vi "Datalog Evaluator.vi"(5 "LuaVIEW reference":T1) -> (15 "error out":errorcluster)   [LabVIEW 2012]
doc: "This plug-in is required by the \"datalogging\" runlevel. It performs tag expression evaluation updates."
uses:
  luaview/typedefs/t_LuaVIEW Reference.ctl
  typedefs/t_Datalog Periodic Evaluator States.ctl
  typedefs/t_DataLog Expression Update Timing Methods.ctl
  typedefs/t_DataLog Tag Info List Methods.ctl
  typedefs/t_DataLog Tag Expression Evaluator Methods.ctl
  luaview/typedefs/t_LuaVIEW Task State Methods.ctl
  luaview/subvis/private/LuaVIEW Pull (flat data).vi
  subvis/private/glb_DataLog Runtime Parameterisation.vi
panel:
  in  "default config":cluster{"tag expression definitions":string}
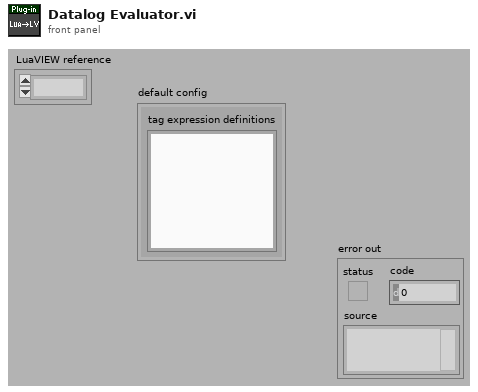
[diagram p1: front panel]
types:
  T1 = typedef "t_LuaVIEW Reference.ctl" = refnum<k1>
  T2 = typedef "t_Datalog Periodic Evaluator States.ctl" = enum16{"empty queue", "poll due tags", "initialize", "init config", "init definitions", "init timing", "init eval", "init active", "cleanup", "stop"}
  T3 = typedef "t_DataLog Expression Update Timing Methods.ctl" = enum16{"initialize", "schedule", "make due", "next due", "cleanup"}
  T4 = typedef "t_DataLog Tag Info List Methods.ctl" = enum16{"initialize", "create", "create empty", "rename", "delete", "test tag", "get", "get by name", "get default", "get list", "get path", "get subsets", "set subsets", "set config", "set capacity", "#tags", "go live", "set unlocked", "set mirrored"}
  T5 = typedef "t_DataLog Tag Expression Evaluator Methods.ctl" = enum16{"set", "get", "eval", "assign", "execute", "isvalid", "clear"}
  T6 = typedef "t_LuaVIEW Task State Methods.ctl" = enum16{"cleanup", "set initial", "set mode", "set active mode", "set error", "get task info", "get script info", "set signal", "clear signal", "test handled", "test delegated", "test signal", "handle signal", "delegate signal", "allow signal", "disallow signal", "disallow all", "signals?", "delegated signals?", "protection++", "protection--", "protection=0", "message", "next message", "pop message", "message available?", "force stop", "set swap preps", "apply swap preps"}
  T7 = typedef "t_DataLog Tag Config.ctl" = cluster{"name":string, "unit":string, "temporal":T8, "value":T9, "index":i32, "capacity":i32, "is meta?":bool, "mincapacity":i32, "deadband":dbl, "limit delay":dbl, "format":T10, "precision":u8, "undefine":bool, "update":bool, "update period":u16, "expression":string, "description":string, "logging algorithm":T11, "logging parameters":dbl[]}
  T8 = typedef "t_DataLog Temporal Types.ctl" = enum16{"set&hold", "sample", "event"}
  T9 = typedef "t_DataLog Value Types.ctl" = enum16{"number", "string"}
  T10 = typedef "t_DataLog Numerical Format.ctl" = enum8{"fractional", "exponential", "engineering"}
  T11 = typedef "t_DataLog Logging Algorithms.ctl" = enum16{"nothing", "changes", "everything", "every Nth", "time threshold", "value threshold + prior", "t or v threshold", "t or v threshold + prior"}
  T12 = typedef "t_LuaVIEW Task State Pane.ctl" = refnum<vi>
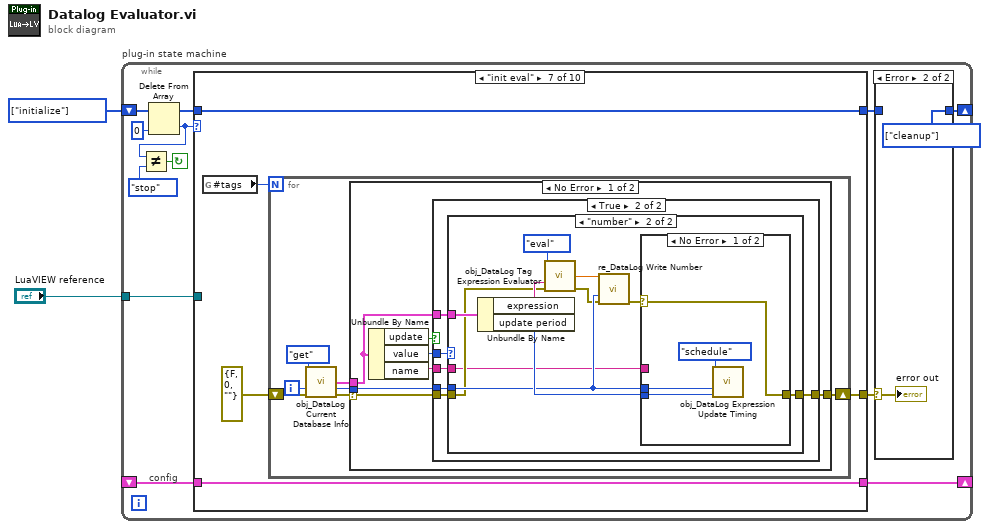
[diagram p0: block diagram]
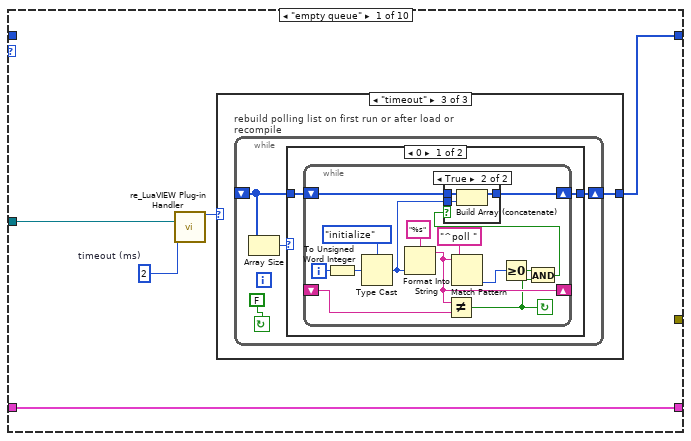
[diagram p3: hidden frame]
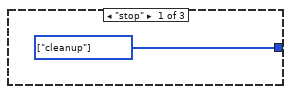
[diagram p4: hidden frame]
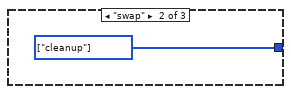
[diagram p5: hidden frame]
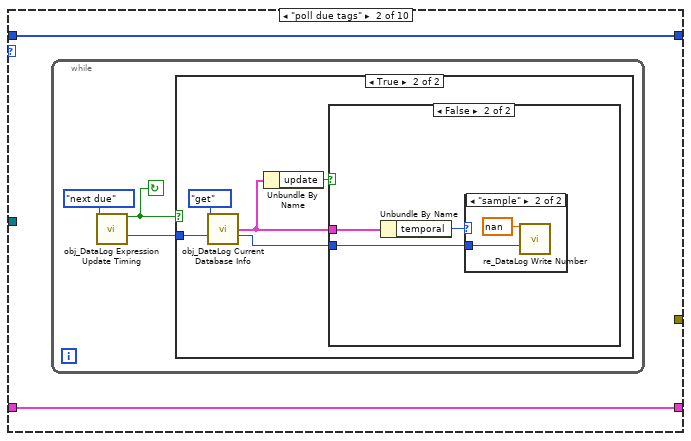
[diagram p8: hidden frame]
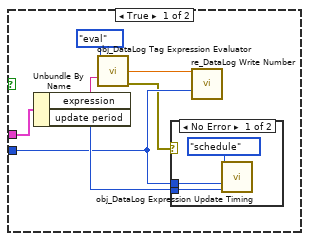
[diagram p10: hidden frame]
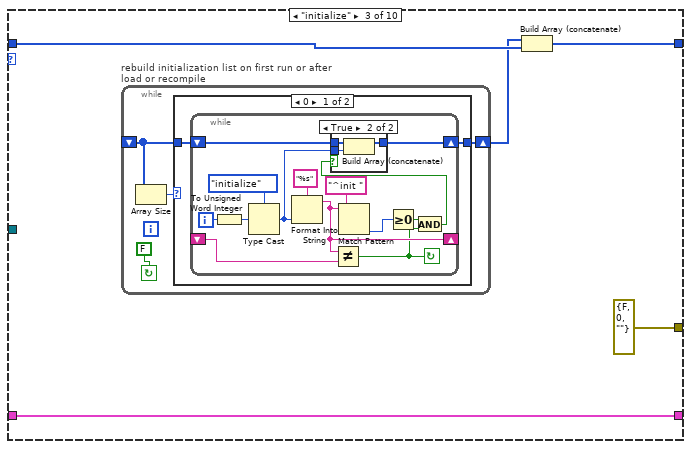
[diagram p13: hidden frame]
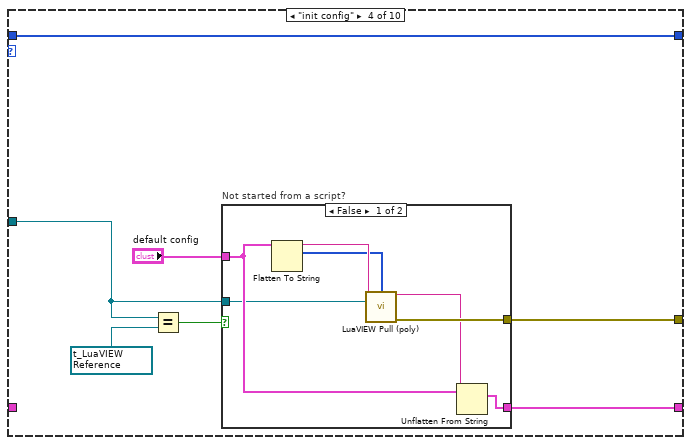
[diagram p16: hidden frame]
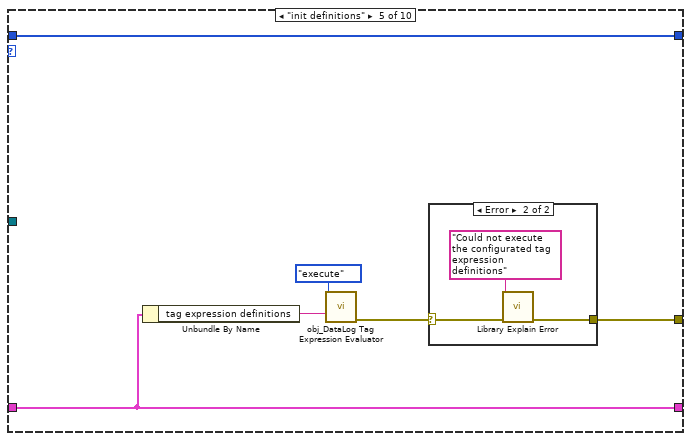
[diagram p18: hidden frame]
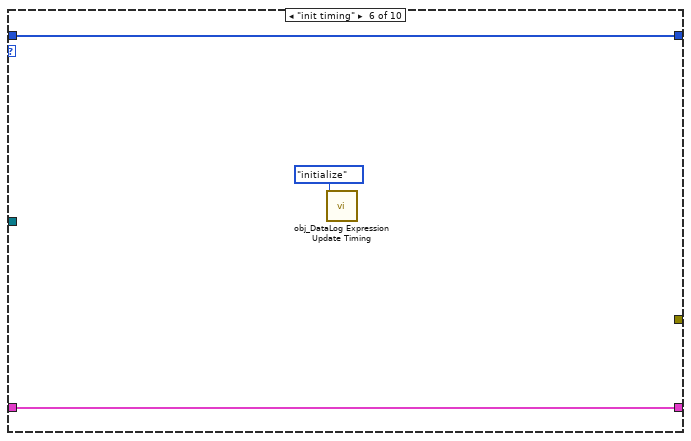
[diagram p20: hidden frame]
diagram:
  w2 = T2[] [enum."initialize"] items=["empty queue", "poll due tags", "initialize", "init config", "init definitions", "init timing", "init eval", "init active", "cleanup", "stop"] ("Array Constant")
  n1 = while "plug-in state machine" {
    shift-left: w2 -> [w12]
    shift-right: [w6] -> _
    tunnel: "LuaVIEW reference" -> [w8]
    shift-right: [w4] -> _
    shift-left: _ -> [w3]
    stop <- w14 continue-if-true
    # "config"
    n2 = Delete From Array(array=w12, index=0) -> (deleted portion=w10:T2, array with subset deleted=w11:T2[])  [unwired: 1 in]
    n3 = Not Equal?(x=w10, y=t_Datalog_Periodic_Evaluator_States."stop" ("states")) -> (x != y?=w14:bool)
    n4 = case "Case" shown="\"init eval\"" w10 {
      tunnel: [w22 w51 w80 w112 w126 w131 w137 w187 w196 w199] -> w7
      tunnel: w11 -> [_ w51 w79 w112 w126 w131 w137 w187 _ w199]
      tunnel: w8 -> [w19 _ _ w107 _ _ _ w188 _ _]
      tunnel: [_ _ errorcluster {"status"=FALSE, "code"=0, "source"=""} ("error out") w111 w124 _ w136 w186 _ _] -> w5
      tunnel: [w18 w52 w77 w109 w123 w133 w138 w191 w197 w198] -> w4
      tunnel: w3 -> [w18 w52 w77 _ w123 w133 w138 w191 w197 w198]
      frame "empty queue" {
        w21 = 2  # timeout (ms)
        n5 = call "re_LuaVIEW Plug-in Handler.vi"("LuaVIEW reference"=w19, "timeout (ms)"=w21) -> ("handle"=w20:enum16{"timeout", "swap", "stop"})  [unwired: 13 in]
        n6 = case shown="\"timeout\"" w20 {
          tunnel: [w23 w24 w25] -> w22
          frame "stop" {
            w23 = T2[] [enum."cleanup"] items=["empty queue", "poll due tags", "initialize", "init config", "init definitions", "init timing", "init eval", "init active", "cleanup", "stop"] ("Array Constant")
          }
          frame "swap" {
            w24 = T2[] [enum."cleanup"] items=["empty queue", "poll due tags", "initialize", "init config", "init definitions", "init timing", "init eval", "init active", "cleanup", "stop"] ("Array Constant")
          }
          frame "timeout" {
            n7 = while "rebuild polling list on first run or after load or recompile" {
              shift-left: _ -> [w28]
              shift-right: [w27] -> w25
              stop <- FALSE continue-if-true
              n8 = Array Size(array=w28) -> (size(s)=w29:i32)
              n9 = case shown="0" w29 {
                tunnel: [w30 w50] -> w27
                tunnel: w28 -> [w31 w50]
                frame 0 {
                  n10 = while {
                    shift-left: w31 -> [w41]
                    shift-right: [w39] -> w30
                    shift-left: _ -> [w42]
                    shift-right: [w38] -> _
                    i -> [w45]
                    stop <- w34 continue-if-true
                    n11 = To Unsigned Word Integer(number=w45) -> (unsigned 16bit integer=w43:u16)
                    n12 = Type Cast(type=t_Datalog_Periodic_Evaluator_States."initialize" ("states"), x=w43) -> (*(type *) &x=w40:T2)
                    n13 = Format Into String(format string="%s" ("Format String"), w40) -> (resulting string=w38:string)  [unwired: 2 in, 1 out]
                    n14 = Not Equal?(x=w38, y=w42) -> (x != y?=w34:bool)
                    n15 = Match Pattern(string=w38, regular expression="^poll ") -> (offset past match=w36:i32)  [unwired: 1 in, 3 out]
                    n16 = Greater Or Equal To 0?(x=w36) -> (x >= 0?=w35:bool)
                    n17 = And(x=w35, y=w34) -> (x .and. y?=w33:bool)
                    n18 = case shown="True" w33 {
                      tunnel: w41 -> [w46 w49]
                      tunnel: w40 -> [_ w48]
                      tunnel: [w46 w47] -> w39
                      frame False {
                      }
                      frame True {
                        n19 = Build Array (concatenate)(w49, w48) -> (w47:T2[])
                      }
                    }
                  }
                }
                frame Default {
                }
              }
            }
          }
        }
      }
      frame "poll due tags" {
        n20 = while {
          stop <- w55 continue-if-true
          n21 = call "obj_DataLog Expression Update Timing.vi"("method"=t_DataLog_Expression_Update_Timing_Methods."next due") -> ("available? {next due}"=w55:bool, "tag index out"=w54:i32)  [unwired: 13 in]
          n22 = case shown="True" w55 {
            tunnel: w54 -> [_ w57]
            frame False {
            }
            frame True {
              n23 = call "obj_DataLog Current Database Info.vi"("method"=t_DataLog_Tag_Info_List_Methods."get", "tag index/change#"=w57) -> ("tag config out"=w58:T7, "dup tag index"=w56:i32)  [unwired: 7 in, 5 out]
              n24 = Unbundle By Name(w58) -> ("update"=w59:bool)
              n25 = case shown="False" w59 {
                tunnel: w58 -> [w67 w72]
                tunnel: w56 -> [w62 w73]
                frame True {
                  n26 = Unbundle By Name(w67) -> ("expression"=w65:string, "update period"=w64:u16)
                  n27 = call "obj_DataLog Tag Expression Evaluator.vi"("method"=t_DataLog_Tag_Expression_Evaluator_Methods."eval", "expression/scriptlet"=w65) -> ("value out"=w63:dbl, "error out"=w61:errorcluster)  [unwired: 12 in]
                  n28 = case shown="No Error" w61 {
                    tunnel: w64 -> [w69 _]
                    tunnel: w62 -> [w68 _]
                    frame No Error {
                      n29 = call "obj_DataLog Expression Update Timing.vi"("method"=t_DataLog_Expression_Update_Timing_Methods."schedule", "tag index"=w68, "period (ms)"=w69) -> ()  [unwired: 11 in, 2 out]
                    }
                    frame Error {
                    }
                  }
                  n30 = call "re_DataLog Write Number.vi"("number"=w63, "tag index in (use tag)"=w62) -> ()  [unwired: 12 in, 2 out]
                }
                frame False {
                  n31 = Unbundle By Name(w72) -> ("temporal"=w71:T8)
                  n32 = case shown="\"sample\"" w71 {
                    tunnel: w73 -> [_ w75]
                    frame "set&hold", Default {
                    }
                    frame "sample" {
                      n33 = call "re_DataLog Write Number.vi"("number"=nan ("value"), "tag index in (use tag)"=w75) -> ()  [unwired: 12 in, 2 out]
                    }
                  }
                }
              }
            }
          }
        }
      }
      frame "initialize" {
        n34 = while "rebuild initialization list on first run or after load or recompile" {
          shift-left: _ -> [w83]
          shift-right: [w82] -> w78
          stop <- FALSE continue-if-true
          n35 = Array Size(array=w83) -> (size(s)=w84:i32)
          n36 = case shown="0" w84 {
            tunnel: [w85 w105] -> w82
            tunnel: w83 -> [w86 w105]
            frame 0 {
              n37 = while {
                shift-left: w86 -> [w95]
                shift-right: [w93] -> w85
                shift-left: _ -> [w97]
                shift-right: [w92] -> _
                i -> [w100]
                stop <- w88 continue-if-true
                n38 = To Unsigned Word Integer(number=w100) -> (unsigned 16bit integer=w98:u16)
                n39 = Type Cast(type=t_Datalog_Periodic_Evaluator_States."initialize" ("states"), x=w98) -> (*(type *) &x=w94:T2)
                n40 = Format Into String(format string="%s" ("Format String"), w94) -> (resulting string=w92:string)  [unwired: 2 in, 1 out]
                n41 = Not Equal?(x=w92, y=w97) -> (x != y?=w88:bool)
                n42 = Match Pattern(string=w92, regular expression="^init ") -> (offset past match=w90:i32)  [unwired: 1 in, 3 out]
                n43 = Greater Or Equal To 0?(x=w90) -> (x >= 0?=w89:bool)
                n44 = And(x=w89, y=w88) -> (x .and. y?=w87:bool)
                n45 = case shown="True" w87 {
                  tunnel: w95 -> [w101 w104]
                  tunnel: w94 -> [_ w103]
                  tunnel: [w101 w102] -> w93
                  frame False {
                  }
                  frame True {
                    n46 = Build Array (concatenate)(w104, w103) -> (w102:T2[])
                  }
                }
              }
            }
            frame Default {
            }
          }
        }
        n47 = Build Array (concatenate)(w78, w79) -> (w80:T2[])
      }
      frame "init config" {
        w108 = T1 refnum items=["LuaVIEW"] ("LuaVIEW reference")
        n48 = Equal?(x=w107, y=w108) -> (x = y?=w106:bool)
        n49 = case "Not started from a script?" shown="False" w106 {
          tunnel: [w119 _] -> w111
          tunnel: "default config" -> [w116 w120]
          tunnel: [w114 w120] -> w109
          tunnel: w107 -> [w113 _]
          frame False {
            n50 = Flatten To String(anything=w116) -> (data string=w118:string, type string=w117:i16[])  [unwired: 3 in, 1 out]
            n51 = call-poly "LuaVIEW Pull (poly).vi"("default flat data"=w118, "type descriptor"=w117, "LuaVIEW reference in"=w113) -> ("flat data"=w115:string, "error out"=w119:errorcluster)  [unwired: 10 in, 1 out]
            n52 = Unflatten From String(type=w116, binary string=w115) -> (value=w114:cluster{"tag expression definitions":string})  [unwired: 3 in, 2 out]
          }
          frame True {
            # "Not relying on a  LuaVIEW state\nallows for testing of the plug-in\nsimply by hitting the run button."
          }
        }
      }
      frame "init definitions" {
        n53 = Unbundle By Name(w123) -> ("tag expression definitions"=w122:string)
        n54 = call "obj_DataLog Tag Expression Evaluator.vi"("method"=t_DataLog_Tag_Expression_Evaluator_Methods."execute", "expression/scriptlet"=w122) -> ("error out"=w121:errorcluster)  [unwired: 12 in, 1 out]
        n55 = case shown="Error" w121 {
          selector: w121 -> [w127 w128]
          tunnel: [w127 w130] -> w124
          frame No Error {
          }
          frame Error {
            n56 = call "Library Explain Error.vi"("explanation prefix (none)"="Could not execute the configurated tag expression definitions", "error in (no error)"=w128) -> ("explained error"=w130:errorcluster)  [unwired: 13 in]
          }
        }
      }
      frame "init timing" {
        n57 = call "obj_DataLog Expression Update Timing.vi"("method"=t_DataLog_Expression_Update_Timing_Methods."initialize") -> ()  [unwired: 13 in, 2 out]
      }
      frame "init eval" {
        n58 = global read "glb_DataLog Runtime Parameterisation.vi" "#tags"() -> (w134:i32)
        n59 = for {
          N: w134 -> [_]
          shift-right: [w145] -> w136
          shift-left: errorcluster {"status"=FALSE, "code"=0, "source"=""} ("error out") -> [w143]
          i -> [w141]
          n60 = call "obj_DataLog Current Database Info.vi"("method"=t_DataLog_Tag_Info_List_Methods."get", "tag index/change#"=w141, "error in (no error)"=w143) -> ("tag config out"=w140:T7, "dup tag index"=w139:i32, "error out"=w142:errorcluster)  [unwired: 6 in, 4 out]
          n61 = case shown="No Error" w142 {
            selector: w142 -> [w147 w185]
            tunnel: w139 -> [w151 _]
            tunnel: [w150 w185] -> w145
            tunnel: w140 -> [w146 _]
            frame No Error {
              n62 = Unbundle By Name(w146) -> ("update"=w152:bool, "value"=w149:T9, "name"=w148:string)
              n63 = case shown="True" w152 {
                tunnel: w146 -> [_ w159]
                tunnel: w151 -> [_ w158]
                tunnel: w147 -> [w153 w157]
                tunnel: [w153 w156] -> w150
                tunnel: w149 -> [_ w155]
                tunnel: w148 -> [_ w154]
                frame False {
                }
                frame True {
                  n64 = case shown="\"number\"" w155 {
                    selector: w155 -> [w162 _]
                    tunnel: w159 -> [_ w175]
                    tunnel: w158 -> [_ w170]
                    tunnel: w157 -> [_ w169]
                    tunnel: [w164 w166] -> w156
                    tunnel: w154 -> [w161 w165]
                    frame "string" {
                      n65 = Format Into String(format string="Cannot update tag \"%s\" by evaluating an expresson: it is a %s tag. The tag has been improperly configured.", w161, w162) -> (resulting string=w160:string)  [unwired: 2 in, 1 out]
                      n66 = call "Library Explain Error.vi"("explanation prefix (none)"=w160) -> ("explained error"=w164:errorcluster)  [unwired: 14 in]
                    }
                    frame "number" {
                      n67 = Unbundle By Name(w175) -> ("expression"=w173:string, "update period"=w172:u16)
                      n68 = call "obj_DataLog Tag Expression Evaluator.vi"("method"=t_DataLog_Tag_Expression_Evaluator_Methods."eval", "expression/scriptlet"=w173, "error in (no error)"=w169) -> ("value out"=w171:dbl, "error out"=w168:errorcluster)  [unwired: 11 in]
                      n69 = call "re_DataLog Write Number.vi"("number"=w171, "tag index in (use tag)"=w170, "error in (no error)"=w168) -> ("error out"=w167:errorcluster)  [unwired: 11 in, 1 out]
                      n70 = case shown="No Error" w167 {
                        selector: w167 -> [w176 w184]
                        tunnel: w172 -> [w178 _]
                        tunnel: w170 -> [w177 _]
                        tunnel: [w176 w183] -> w166
                        tunnel: w165 -> [_ w181]
                        frame No Error {
                          n71 = call "obj_DataLog Expression Update Timing.vi"("method"=t_DataLog_Expression_Update_Timing_Methods."schedule", "tag index"=w177, "period (ms)"=w178) -> ()  [unwired: 11 in, 2 out]
                        }
                        frame Error {
                          n72 = Format Into String(format string="The initial evaluation of tag \"%s\" failed. The configured tag expression is likely invalid.", w181) -> (resulting string=w180:string)  [unwired: 2 in, 1 out]
                          n73 = call "Library Explain Error.vi"("explanation prefix (none)"=w180, "error in (no error)"=w184) -> ("explained error"=w183:errorcluster)  [unwired: 13 in]
                        }
                      }
                    }
                  }
                }
              }
            }
            frame Error {
            }
          }
        }
      }
      frame "init active" {
        n74 = call "LuaVIEW Get Task State Reference.vi"("LuaVIEW reference in"=w188) -> ("task state reference"=w189:T12, "error out"=w190:errorcluster)  [unwired: 12 in, 1 out]
        n75 = case "a task?" shown="No Error" w190 {
          tunnel: w189 -> [w193 _]
          tunnel: [w192 _] -> w186
          frame No Error {
            # "We've made it through the initialization.\nActivate the task so as to complete\ndeferred initialization."
            n76 = call-by-ref "?"(reference=w193, "method"=t_LuaVIEW_Task_State_Methods."set active mode") -> (error out=w192:errorcluster)  [unwired: 11 in, 6 out]
          }
          frame Error {
          }
        }
      }
      frame "cleanup" {
        w196 = T2[] [enum."stop"] items=["empty queue", "poll due tags", "initialize", "init config", "init definitions", "init timing", "init eval", "init active", "cleanup", "stop"] ("Array Constant")
        n77 = call "obj_DataLog Expression Update Timing.vi"("method"=t_DataLog_Expression_Update_Timing_Methods."cleanup") -> ()  [unwired: 13 in, 2 out]
      }
      frame "stop" {
      }
    }
    n78 = case shown="Error" w5 {
      selector: w5 -> [_ w16]
      tunnel: w7 -> [w15 _]
      tunnel: [w15 w17] -> w6
      frame No Error {
      }
      frame Error {
        w17 = T2[] [enum."cleanup"] items=["empty queue", "poll due tags", "initialize", "init config", "init definitions", "init timing", "init eval", "init active", "cleanup", "stop"] ("Array Constant")
        "error out" <- w16
      }
    }
  }
